vi "MeasurementServer_SetResponse_FourProbeMeasurement.vi"(0 "gRPCid":T4, 1 "FourProbeResponse":T1, 3 "error in (no error)":errorcluster) -> (10 "error out":errorcluster)   [LabVIEW 2019, in "labview-grpc-measurement-server.lvlib"]
uses:
  labview-grpc-measurement-server.lvlib
  MeasurementServer_gRPCid.ctl
  MeasurementServer_FourProbeResponse.ctl
  MeasurementServer_FourProbeRawData.ctl
  MeasurementServer_ErrorOutData.ctl
  build/Debug/labview_measurement_server.dll
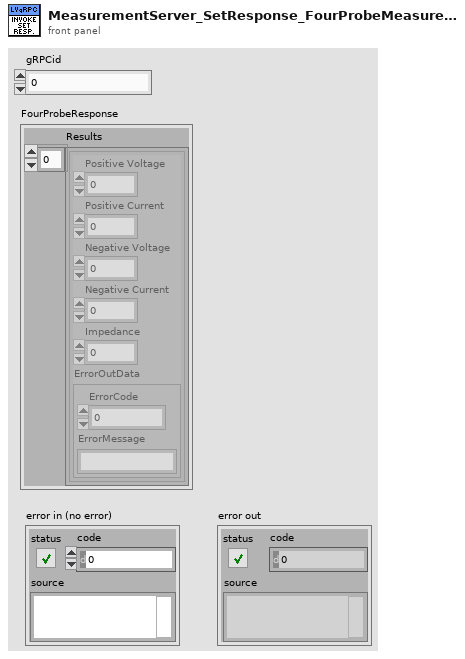
[diagram p1: front panel]
types:
  T1 = typedef "labview-grpc-measurement-server.lvlib/MeasurementServer_FourProbeResponse.ctl" = cluster{"Results":T2[]}
  T2 = typedef "labview-grpc-measurement-server.lvlib/MeasurementServer_FourProbeRawData.ctl" = cluster{"Positive Voltage":sgl, "Positive Current":sgl, "Negative Voltage":sgl, "Negative Current":sgl, "Impedance":sgl, "ErrorOutData":T3}
  T3 = typedef "labview-grpc-measurement-server.lvlib/MeasurementServer_ErrorOutData.ctl" = cluster{"ErrorCode":i32, "ErrorMessage":string}
  T4 = typedef "labview-grpc-measurement-server.lvlib/MeasurementServer_gRPCid.ctl" = u64
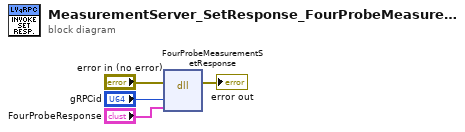
[diagram p0: block diagram]
diagram:
  n1 = dll-call lib="C:/dev/labview-grpc-measurement-server/build/Debug/labview_measurement_server.dll" fn="FourProbeMeasurementSetResponse"(error in="error in (no error)", "id"="gRPCid", "data"="FourProbeResponse") -> (error out=→"error out":errorcluster)  [unwired: 5 in, 1 out]
